vi "标签导出.vi"(8 "error in":errorcluster caption="错误输入（无错误）", 9 "目标仓库":path, 10 "标签（版本）":string, 11 "仓库路径":path) -> (0 "error out":errorcluster caption="错误输出", 1 "standard error":string caption="标准错误", 2 "standard output":string caption="标准输出", 3 "仓库路径":path)   [LabVIEW 2018]
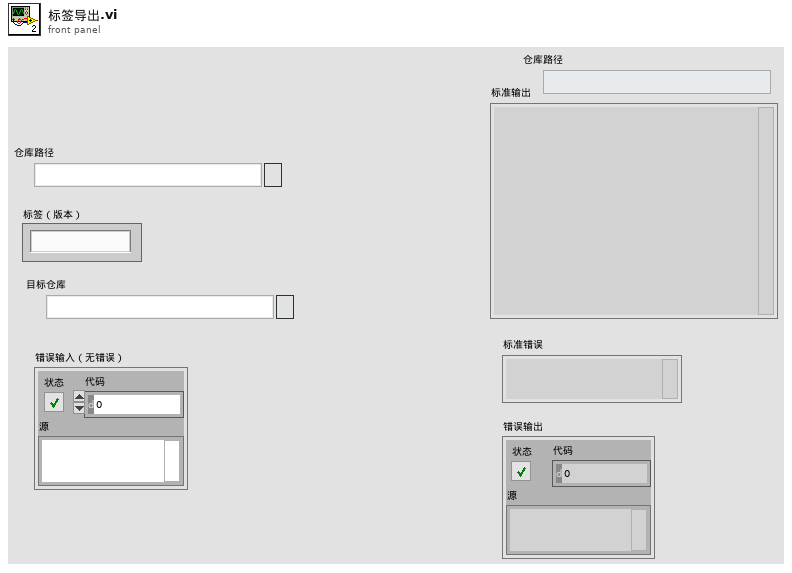
[diagram p1: front panel]
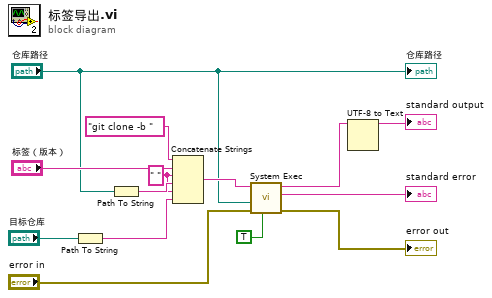
[diagram p0: block diagram]
diagram:
  w3 = " " ("字符串")
  n1 = Path To String(path="目标仓库") -> (string=w1:string)
  n2 = Path To String(path="仓库路径") -> (string=w4:string)
  n3 = Concatenate Strings("git clone -b " ("command line"), "标签（版本）", w3, w4, w3, w1) -> (w7:string)
  n4 = call <vilib>:"System Exec.vi"("run minimized? (F)"=TRUE, "error in (no error)"="error in", "working directory"="仓库路径", "command line"=w7) -> ("error out"=→"error out":errorcluster, "standard error"=→"standard error":string, "standard output"=w13:string)  [unwired: 4 in, 1 out]
  n5 = UTF-8 to Text ("UTF-8至文本转换")(11:w13) -> (3:→"standard output":string)  [unwired: 2 in, 1 out]
  "仓库路径" <- "仓库路径"
